vi "Memory.Pointer.Read Bytes.Subset.In Place.Safe.vi"(7 "length":u64 format="%d bytes", 8 "error in (no error)":errorcluster, 9 "offset (0)":u64 format="%d bytes", 10 "buffer in":u8[](array[numeric]) format="%02x", 11 "Pointer in":refnum<class "Memory.Pointer.Void.lvclass">) -> (0 "error out":errorcluster, 1 "offset dup":u64 format="%d bytes", 2 "buffer out":u8[](array[numeric]) format="%02x", 3 "Pointer out":refnum<class "Memory.Pointer.Void.lvclass">)   [LabVIEW 2016, in "LabVIEW Memory Manager.lvlib" / "Memory.Pointer.Void.lvclass"]
uses:
  Memory.Pointer.Void.lvclass
  Memory.Pointer.Void.lvclass/Memory.Pointer.Void.ctl
  Memory.Pointer.Get Size.vi
  Memory.Pointer.Parameter Check.Length.vi
  Memory.Pointer.Parameter Check.Offset.vi
  Memory.Pointer.Offset to Address.vi
  Memory.Pointer.Offset to Address.Unsafe.vi
  Memory.Pointer.Get Address.vi
  Memory.Pointer.Error Handling.Out of Range.vi
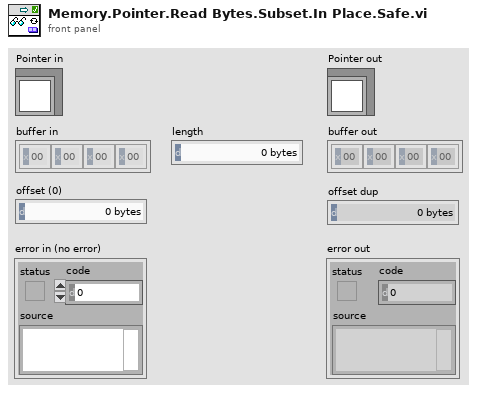
[diagram p1: front panel]
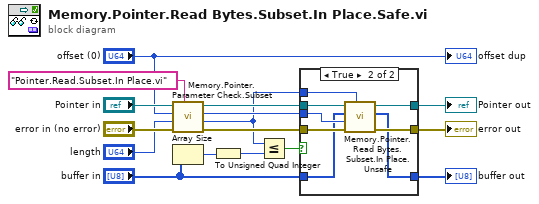
[diagram p0: block diagram]
diagram:
  n1 = call "Memory.Pointer.Parameter Check.Subset.vi"("calling vi name"="Pointer.Read.Subset.In Place.vi", "error in (no error)"="error in (no error)", "length"="length", "offset"="offset (0)", "Pointer in"="Pointer in") -> ("error out"=w7:errorcluster, "length out"=w3:u64, "offset out"=w5:u64, "Pointer out"=w8:refnum<class "Memory.Pointer.Void.lvclass">)  [unwired: 3 in]
  n2 = Array Size(array="buffer in") -> (size(s)=w14:i32)
  n3 = To Unsigned Quad Integer(1:w14) -> (0:w6:u64)
  n4 = Less Or Equal?(x=w3, y=w6) -> (x <= y?=w2:bool)
  n5 = case shown="True" w2 {
    tunnel: [w19 w26] -> w16
    tunnel: [w18 w23] -> w15
    tunnel: [w17 w22] -> w10
    tunnel: w8 -> [w19 w27]
    tunnel: w7 -> [w18 w24]
    tunnel: w5 -> [_ w21]
    tunnel: "buffer in" -> [w17 w20]
    tunnel: w3 -> [_ w25]
    frame False {
      # "#TODO\nThrow error."
    }
    frame True {
      n6 = call "Memory.Pointer.Read Bytes.Subset.In Place.Unsafe.vi"("length"=w25, "error in (no error)"=w24, "offset (0)"=w21, "buffer in"=w20, "Pointer in"=w27) -> ("error out"=w23:errorcluster, "buffer out"=w22:u8[], "Pointer out"=w26:refnum<class "Memory.Pointer.Void.lvclass">)  [unwired: 3 in, 1 out]
    }
  }
  "error out" <- w15
  "Pointer out" <- w16
  "buffer out" <- w10
  "offset dup" <- "offset (0)"
